vi "主程序.vi"() -> ()   [LabVIEW 2010]
panel:
  out "z_fomula":dbl
  out "z_case":dbl
  in  "y":dbl
  in  "x":dbl
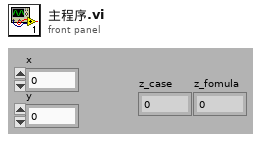
[diagram p1: front panel]
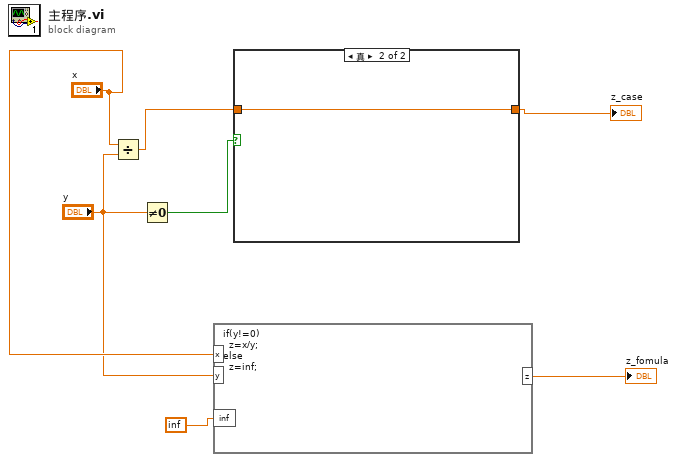
[diagram p0: block diagram]
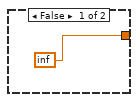
[diagram p2: hidden frame]
diagram:
  n1 = Divide(x="x", y="y") -> (x/y=w6:dbl)
  n2 = Not Equal To 0?(x="y") -> (x != 0?=w7:bool)
  n3 = formula code="if(y!=0)\n  z=x/y;\nelse\n  z=inf;"("x"="x", "y"="y", "inf"=inf) -> ("z"=→"z_fomula":dbl)
  n4 = case shown="真" w7 {
    tunnel: w6 -> [_ w9]
    tunnel: [inf w9] -> w3
    frame False {
    }
    frame True {
    }
  }
  "z_case" <- w3
